vi "I2S Index (David Documentation).vi"(8 "Bit Count":u16=32 max=32, 9 "Update":bool, 10 "Change Channel":bool) -> (3 "Value Out":u16=32)   [LabVIEW 2015]
panel:
  # "Overview: Generate bitwise index of digital audio data."
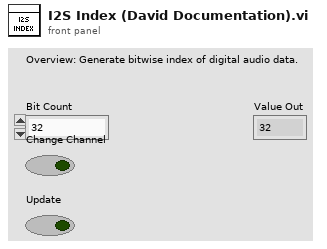
[diagram p1: front panel]
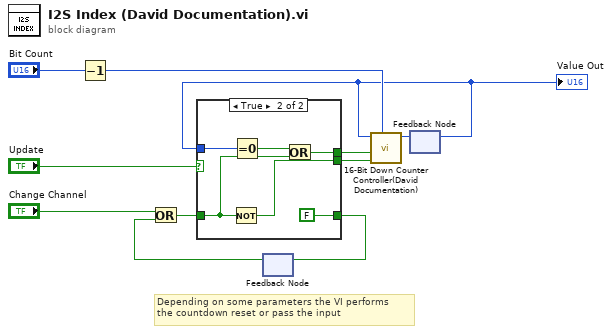
[diagram p0: block diagram]
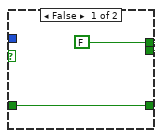
[diagram p2: hidden frame]
diagram:
  # "Depending on some parameters the VI performs \nthe countdown reset or pass the input"
  n1 = Decrement(x="Bit Count") -> (x-1=w10:u16)
  n2 = feedback #1() -> (w4:bool)  [unwired: 1 in]
  n3 = Or(x="Change Channel", y=w4) -> (x .or. y?=w2:bool)
  n4 = feedback #2() -> (w1:u16)  [unwired: 1 in]
  "Value Out" <- w1
  n5 = case shown="True" "Update" {
    tunnel: [w12 w18] -> w8
    tunnel: [w12 w17] -> w7
    tunnel: w1 -> [_ w16]
    tunnel: [w13 FALSE ("t")] -> w3
    tunnel: w2 -> [w13 w14]
    frame False {
      w12 = FALSE
    }
    frame True {
      n6 = Not(x=w14) -> (.not. x?=w17:bool)
      n7 = Equal To 0?(x=w16) -> (x = 0?=w19:bool)
      n8 = Or(x=w19, y=w14) -> (x .or. y?=w18:bool)
    }
  }
  n9 = feedback-in #1(w3) -> ()
  n10 = call "16-Bit Down Counter Controller(David Documentation).vi"("Input"=w10, "Decrement"=w7, "Load"=w8, "Value"=w1) -> ("Value+"=w9:u16)  [unwired: 7 in]
  n11 = feedback-in #2(w9) -> ()
